vi "Init Controller.vi"(10 "CAN Offset":u32 format="%x", 11 "CANTXQueueIn":T1) -> (3 "CANTXQueueOut":T1)   [LabVIEW 2015]
uses:
  TX Library/CAN Message Queue.ctl
  TX Library/CAN Message.ctl
  <vilib>/RioEmbeddedCAN/RioEmbeddedCAN.llb/CANFrameControl.ctl
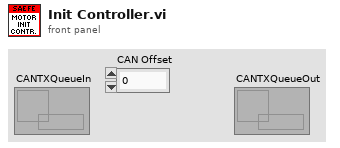
[diagram p1: front panel]
types:
  T1 = typedef "CAN Message Queue.ctl" = refnum<k33>
  T2 = typedef "CANFrameControl.ctl" = cluster{"identifier":u32, "extended?":bool, "type":u8, "payload":u8[]}
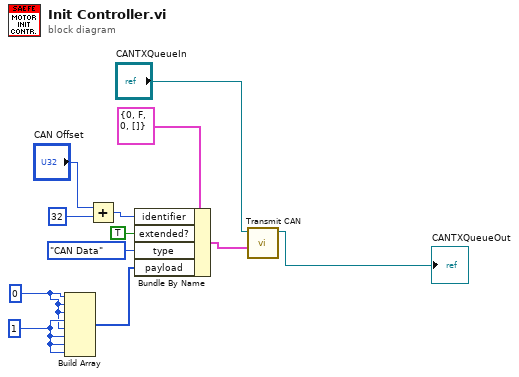
[diagram p0: block diagram]
diagram:
  w5 = u8 1 ("element")
  w4 = u8 0
  n1 = Build Array(w4, w4, w4, w5, w4, w5, w5, w5) -> (w9:u8[])
  n2 = Add(x="CAN Offset", y=u32 32 ("identifier")) -> (x+y=w7:u32)
  n3 = Bundle By Name(cluster=T2 {"identifier"=0, "extended?"=FALSE, "type"=0, "payload"=[]} ("CAN frame"), "identifier"=w7, "extended?"=TRUE, "type"=enum8{"CAN Data", "CAN Remote"}."CAN Data", "payload"=w9) -> (w3:T2)
  n4 = call "Transmit CAN.vi"("CAN Queue"="CANTXQueueIn", "CAN frame"=w3) -> ("CAN Queue Out"=→"CANTXQueueOut":T1)  [unwired: 8 in]
